vi "input to tag bus.vi"(9 "indices":T1, 10 "data cluster":T2 {"AILimitLow" format="%.0x"; "AILimitHigh" format="%.0x"}, 11 "tag bus in":T3) -> (3 "tag bus out":T3)   [LabVIEW 2015, in "GPIC ScaleAndLimit runtime.lvclass"]
uses:
  GPIC ScaleAndLimit runtime.lvclass
  <vilib>/NI/Tag Bus/table/data table.ctl
  input user data.ctl
  configuration/input data indices.ctl
  <vilib>/NI/Tag Bus/table/data polymorphs/write one/write U16.vi
  <vilib>/NI/Tag Bus/table/data polymorphs/write one/write Boolean.vi
  <vilib>/NI/Tag Bus/table/data polymorphs/write one/write Single.vi
  <vilib>/NI/Tag Bus/table/data table.lvlib
  configuration/GPIC ScaleAndLimit configuration.lvclass
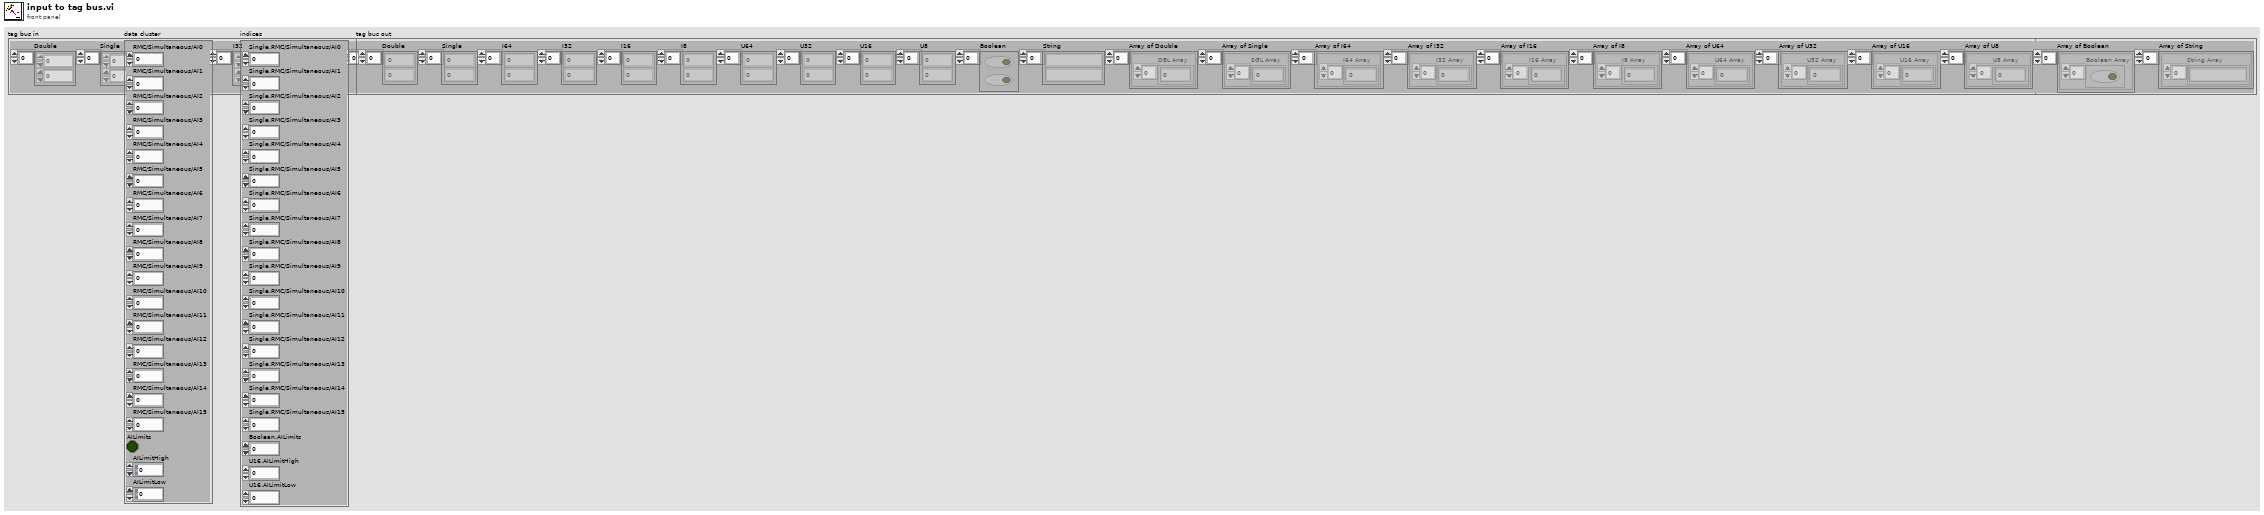
[diagram p1: front panel]
types:
  T1 = typedef "GPIC ScaleAndLimit configuration.lvclass/input data indices.ctl" = cluster{"Single.RMC/Simultaneous/AI0":i32, "Single.RMC/Simultaneous/AI1":i32, "Single.RMC/Simultaneous/AI2":i32, "Single.RMC/Simultaneous/AI3":i32, "Single.RMC/Simultaneous/AI4":i32, "Single.RMC/Simultaneous/AI5":i32, "Single.RMC/Simultaneous/AI6":i32, "Single.RMC/Simultaneous/AI7":i32, "Single.RMC/Simultaneous/AI8":i32, "Single.RMC/Simultaneous/AI9":i32, "Single.RMC/Simultaneous/AI10":i32, "Single.RMC/Simultaneous/AI11":i32, "Single.RMC/Simultaneous/AI12":i32, "Single.RMC/Simultaneous/AI13":i32, "Single.RMC/Simultaneous/AI14":i32, "Single.RMC/Simultaneous/AI15":i32, "Boolean.AILimits":i32, "U16.AILimitHigh":i32, "U16.AILimitLow":i32}
  T2 = typedef "GPIC ScaleAndLimit runtime.lvclass/input user data.ctl" = cluster{"RMC/Simultaneous/AI0":sgl, "RMC/Simultaneous/AI1":sgl, "RMC/Simultaneous/AI2":sgl, "RMC/Simultaneous/AI3":sgl, "RMC/Simultaneous/AI4":sgl, "RMC/Simultaneous/AI5":sgl, "RMC/Simultaneous/AI6":sgl, "RMC/Simultaneous/AI7":sgl, "RMC/Simultaneous/AI8":sgl, "RMC/Simultaneous/AI9":sgl, "RMC/Simultaneous/AI10":sgl, "RMC/Simultaneous/AI11":sgl, "RMC/Simultaneous/AI12":sgl, "RMC/Simultaneous/AI13":sgl, "RMC/Simultaneous/AI14":sgl, "RMC/Simultaneous/AI15":sgl, "AILimits":bool, "AILimitHigh":u16, "AILimitLow":u16}
  T3 = typedef "tag bus.lvlib/data table.lvlib/data table.ctl" = cluster{"Double":dbl[], "Single":sgl[], "I64":i64[], "I32":i32[], "I16":i16[], "I8":i8[], "U64":u64[], "U32":u32[], "U16":u16[], "U8":u8[], "Boolean":bool[], "String":string[], "Array of Double":cluster{"DBL Array":dbl[]}[], "Array of Single":cluster{"SGL Array":sgl[]}[], "Array of I64":cluster{"I64 Array":i64[]}[], "Array of I32":cluster{"I32 Array":i32[]}[], "Array of I16":cluster{"I16 Array":i16[]}[], "Array of I8":cluster{"I8 Array":i8[]}[], "Array of U64":cluster{"U64 Array":u64[]}[], "Array of U32":cluster{"U32 Array":u32[]}[], "Array of U16":cluster{"U16 Array":u16[]}[], "Array of U8":cluster{"U8 Array":u8[]}[], "Array of Boolean":cluster{"Boolean Array":bool[]}[], "Array of String":cluster{"String Array":string[]}[]}
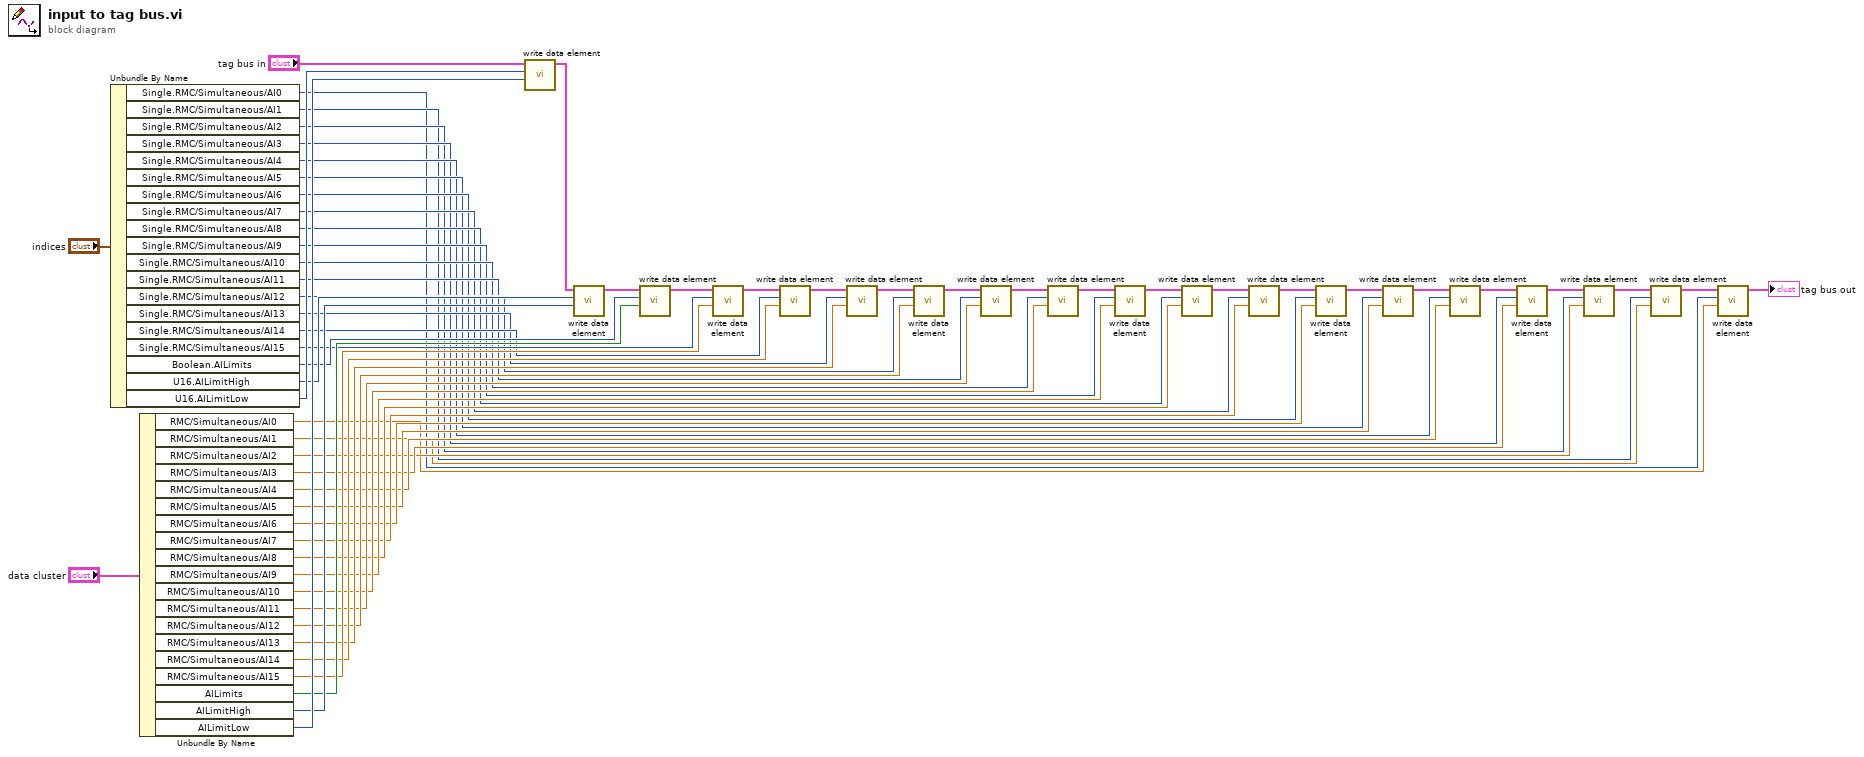
[diagram p0: block diagram]
diagram:
  n1 = Unbundle By Name("indices") -> ("Single.RMC/Simultaneous/AI0"=w4:i32, "Single.RMC/Simultaneous/AI1"=w7:i32, "Single.RMC/Simultaneous/AI2"=w10:i32, "Single.RMC/Simultaneous/AI3"=w13:i32, "Single.RMC/Simultaneous/AI4"=w16:i32, "Single.RMC/Simultaneous/AI5"=w19:i32, "Single.RMC/Simultaneous/AI6"=w22:i32, "Single.RMC/Simultaneous/AI7"=w25:i32, "Single.RMC/Simultaneous/AI8"=w28:i32, "Single.RMC/Simultaneous/AI9"=w31:i32, "Single.RMC/Simultaneous/AI10"=w34:i32, "Single.RMC/Simultaneous/AI11"=w37:i32, "Single.RMC/Simultaneous/AI12"=w40:i32, "Single.RMC/Simultaneous/AI13"=w43:i32, "Single.RMC/Simultaneous/AI14"=w46:i32, "Single.RMC/Simultaneous/AI15"=w49:i32, "Boolean.AILimits"=w52:i32, "U16.AILimitHigh"=w55:i32, "U16.AILimitLow"=w58:i32)
  n2 = Unbundle By Name("data cluster") -> ("RMC/Simultaneous/AI0"=w3:sgl, "RMC/Simultaneous/AI1"=w6:sgl, "RMC/Simultaneous/AI2"=w9:sgl, "RMC/Simultaneous/AI3"=w12:sgl, "RMC/Simultaneous/AI4"=w15:sgl, "RMC/Simultaneous/AI5"=w18:sgl, "RMC/Simultaneous/AI6"=w21:sgl, "RMC/Simultaneous/AI7"=w24:sgl, "RMC/Simultaneous/AI8"=w27:sgl, "RMC/Simultaneous/AI9"=w30:sgl, "RMC/Simultaneous/AI10"=w33:sgl, "RMC/Simultaneous/AI11"=w36:sgl, "RMC/Simultaneous/AI12"=w39:sgl, "RMC/Simultaneous/AI13"=w42:sgl, "RMC/Simultaneous/AI14"=w45:sgl, "RMC/Simultaneous/AI15"=w48:sgl, "AILimits"=w51:bool, "AILimitHigh"=w54:u16, "AILimitLow"=w57:u16)
  n3 = call-poly <vilib>:"write data element.vi"("value"=w57, "index"=w58, "data table in"="tag bus in") -> ("data table out"=w53:T3)  [unwired: 8 in]
  n4 = call-poly <vilib>:"write data element.vi"("value"=w54, "index"=w55, "data table in"=w53) -> ("data table out"=w50:T3)  [unwired: 8 in]
  n5 = call-poly <vilib>:"write data element.vi"("value"=w51, "index"=w52, "data table in"=w50) -> ("data table out"=w47:T3)  [unwired: 8 in]
  n6 = call-poly <vilib>:"write data element.vi"("value"=w48, "index"=w49, "data table in"=w47) -> ("data table out"=w44:T3)  [unwired: 8 in]
  n7 = call-poly <vilib>:"write data element.vi"("value"=w45, "index"=w46, "data table in"=w44) -> ("data table out"=w41:T3)  [unwired: 8 in]
  n8 = call-poly <vilib>:"write data element.vi"("value"=w42, "index"=w43, "data table in"=w41) -> ("data table out"=w38:T3)  [unwired: 8 in]
  n9 = call-poly <vilib>:"write data element.vi"("value"=w39, "index"=w40, "data table in"=w38) -> ("data table out"=w35:T3)  [unwired: 8 in]
  n10 = call-poly <vilib>:"write data element.vi"("value"=w36, "index"=w37, "data table in"=w35) -> ("data table out"=w32:T3)  [unwired: 8 in]
  n11 = call-poly <vilib>:"write data element.vi"("value"=w33, "index"=w34, "data table in"=w32) -> ("data table out"=w29:T3)  [unwired: 8 in]
  n12 = call-poly <vilib>:"write data element.vi"("value"=w30, "index"=w31, "data table in"=w29) -> ("data table out"=w26:T3)  [unwired: 8 in]
  n13 = call-poly <vilib>:"write data element.vi"("value"=w27, "index"=w28, "data table in"=w26) -> ("data table out"=w23:T3)  [unwired: 8 in]
  n14 = call-poly <vilib>:"write data element.vi"("value"=w24, "index"=w25, "data table in"=w23) -> ("data table out"=w20:T3)  [unwired: 8 in]
  n15 = call-poly <vilib>:"write data element.vi"("value"=w21, "index"=w22, "data table in"=w20) -> ("data table out"=w17:T3)  [unwired: 8 in]
  n16 = call-poly <vilib>:"write data element.vi"("value"=w18, "index"=w19, "data table in"=w17) -> ("data table out"=w14:T3)  [unwired: 8 in]
  n17 = call-poly <vilib>:"write data element.vi"("value"=w15, "index"=w16, "data table in"=w14) -> ("data table out"=w11:T3)  [unwired: 8 in]
  n18 = call-poly <vilib>:"write data element.vi"("value"=w12, "index"=w13, "data table in"=w11) -> ("data table out"=w8:T3)  [unwired: 8 in]
  n19 = call-poly <vilib>:"write data element.vi"("value"=w9, "index"=w10, "data table in"=w8) -> ("data table out"=w5:T3)  [unwired: 8 in]
  n20 = call-poly <vilib>:"write data element.vi"("value"=w6, "index"=w7, "data table in"=w5) -> ("data table out"=w2:T3)  [unwired: 8 in]
  n21 = call-poly <vilib>:"write data element.vi"("value"=w3, "index"=w4, "data table in"=w2) -> ("data table out"=→"tag bus out":T3)  [unwired: 8 in]
